vi "Job.BuildSpec_CleanPreviousBuild.vi"(8 "error in (no error)":errorcluster, 11 "Job.BuildSpec in":refnum<class "Job.BuildSpec.lvclass">) -> (0 "error out":errorcluster, 3 "Job.BuildSpec out":refnum<class "Job.BuildSpec.lvclass">)   [LabVIEW 2013, in "Job.BuildSpec.lvclass"]
uses:
  Job.BuildSpec.lvclass
  Job.BuildSpec.lvclass/Job.BuildSpec.ctl
  <vilib>/AppBuilder/AB_API_Simple/NI_App_Builder_API.lvlib
  <vilib>/LabVIEW Open Source Project/Cron Scheduler/Job/Job.lvclass
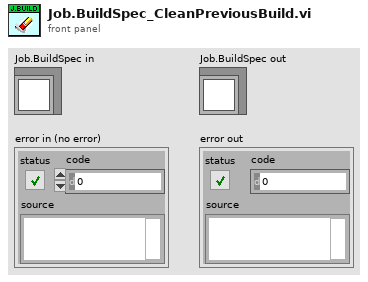
[diagram p1: front panel]
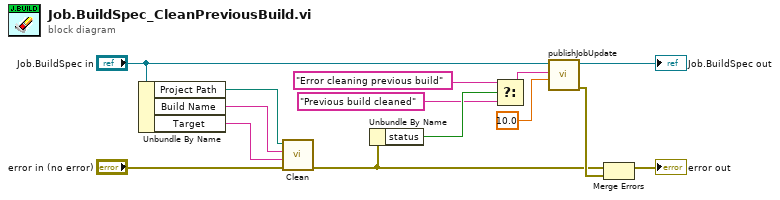
[diagram p0: block diagram]
diagram:
  n1 = Unbundle By Name("Job.BuildSpec in") -> ("Project Path"=w8:path, "Build Name"=w7:string, "Target"=w9:string)
  n2 = call <vilib>:"Clean.vi"("error in (no error)"="error in (no error)", "Name of target (My Computer)"=w9, "Name of build specification (if empty: clean all)"=w7, "Path to project"=w8) -> ("error out"=w2:errorcluster)  [unwired: 7 in]
  n3 = Unbundle By Name(w2) -> ("status"=w5:bool)
  n4 = Select(t="Error cleaning previous build" ("Status Message"), s=w5, f="Previous build cleaned" ("Status Message")) -> (s? t:f=w1:string)
  n5 = call <vilib>:"publishJobUpdate.vi"("% Complete (NaN if unknown)"=10.0, "Status Message"=w1, "Job in"="Job.BuildSpec in") -> ("error out"=w13:errorcluster, "Job out"=→"Job.BuildSpec out":refnum<class "Job.BuildSpec.lvclass">)  [unwired: 7 in]
  n6 = Merge Errors(w2, w13) -> (→"error out":errorcluster)
